vi "GraphForm (SubVI) P.vi"() -> ()   [LabVIEW 2013]
uses:
  Global P.vi
panel:
  out "Sensor 2":dbl format="%.3e"
  out "Sensor 1":dbl format="%.3e"
  in  "P loc":cluster{" P sens 1":dbl, "P sens 2":dbl}
  in  "1_ch_v":bool=TRUE
  in  "stop":bool
  in  "Title":string
  out "часы":string="0"
  in  "Добавить время":dbl(ring)=300.0 items=["1 мин."=60.0, "5 мин."=300.0, "20 мин."=1200.0]
  out "мин.":string="1"
  in  "xScale +":bool
  in  "xScale -":bool
  in  "Autoscale":bool=TRUE
  in  "P max":dbl=0.01 format="%^#.6e"
  in  "P min":dbl=1e-09 format="%^#.6e"
  in  "2_ch_v":bool=TRUE
  in  "T1_col":u32(colorbox)=16448250
  in  "T2_col":u32(colorbox)=2132224
  out "Graphs P":dynamicdata(graph)
  # "P"
  # "[mBar]"
  # "Интервал просмотра"
  # ":"
  # "Шкала P"
  # "P, mBar"
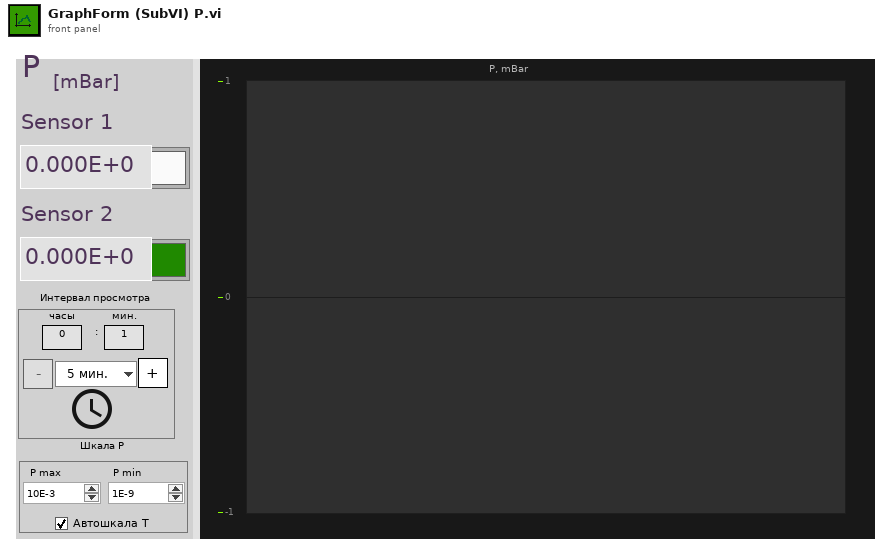
[diagram p1: front panel]
types:
  T1 = typedef "LVDateTimeRec.ctl" = cluster{"fractional second":dbl, "second":i32, "minute":i32, "hour":i32, "day of month":i32, "month":i32, "year":i32, "day of week":i32, "day of year":i32, "DST":i32}
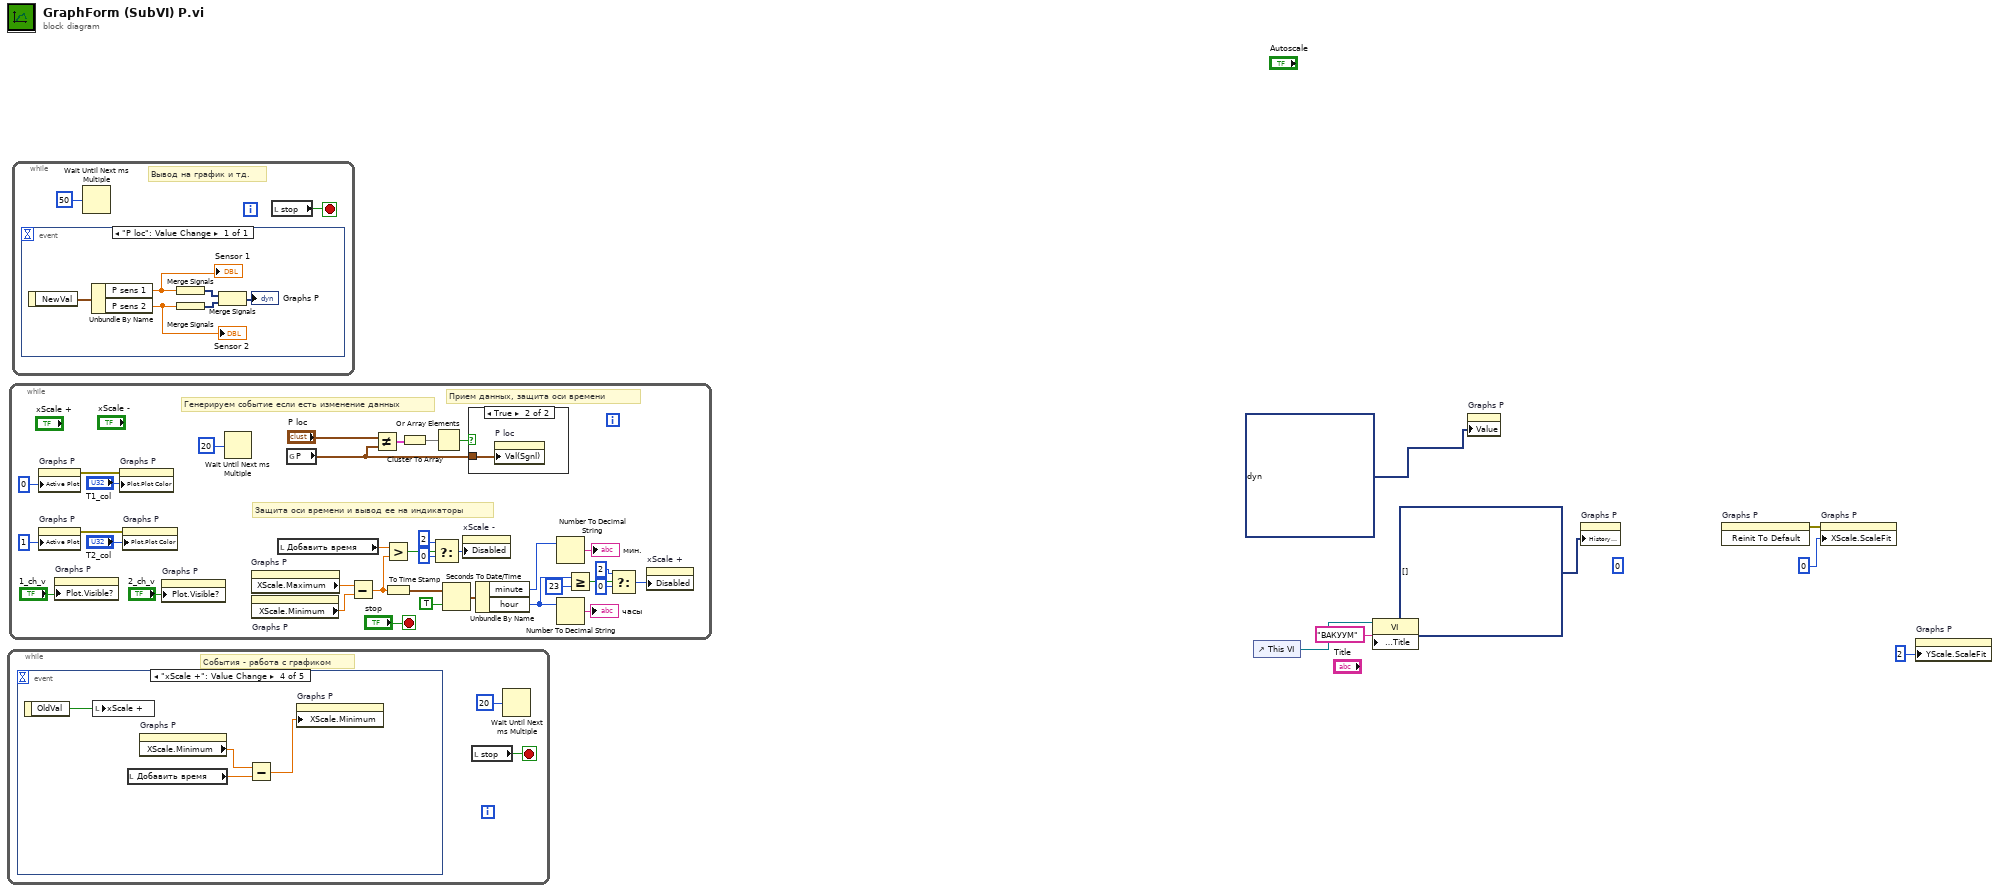
[diagram p0: block diagram]
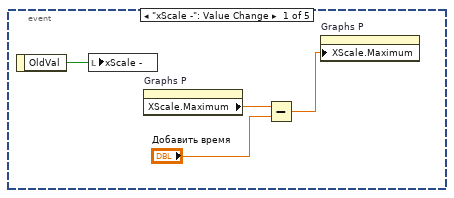
[diagram p3: hidden frame]
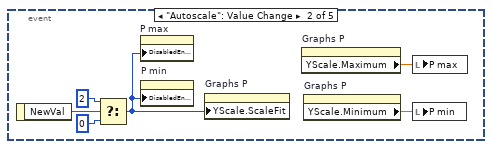
[diagram p4: hidden frame]
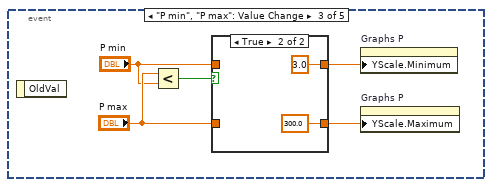
[diagram p5: hidden frame]
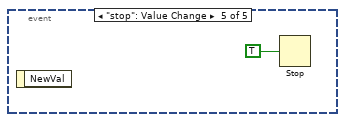
[diagram p7: hidden frame]
diagram:
  (unwired) u8 0 ("Y Scale.Scale Fit")
  n1 = while {
    stop <- w8 stop-if-true
    # "События - работа с графиком"
    n2 = event shown="[3] \"xScale +\": Value Change" {
      selector: _ -> [_ _ _ _ _]
      dyn-events: _ -> [_ _ _ _ _]
      timeout: _ -> [_ _ _ _ _]
      event "xScale -": Value Change {
        n3 = event-data() -> ("OldVal"=w13:bool)  [unwired: 1 out]
        n4 = local write "xScale -"(w13) -> ()
        n5 = property on="Graphs P" class="WFChart (strict)"() -> ("XScale.Maximum"=w11:dbl)  [unwired: 2 in, 2 out]
        n6 = Subtract(x=w11, y="Добавить время") -> (x-y=w12:dbl)
        n7 = property on="Graphs P" class="WFChart (strict)"("XScale.Maximum"=w12) -> ()  [unwired: 2 in, 2 out]
      }
      event "Autoscale": Value Change {
        n8 = event-data() -> ("NewVal"=w14:bool)  [unwired: 1 out]
        n9 = Select(t=u8 2 ("Y Scale.Scale Fit"), s=w14, f=u8 0 ("Y Scale.Scale Fit")) -> (s? t:f=w17:u8)
        n10 = property on="P max" class="DigNum (strict)"("DisabledEnum"=w17) -> ()  [unwired: 2 in, 2 out]
        n11 = property on="P min" class="DigNum (strict)"("DisabledEnum"=w17) -> ()  [unwired: 2 in, 2 out]
        n12 = property on="Graphs P" class="WFChart (strict)"("YScale.ScaleFit"=w17) -> ()  [unwired: 2 in, 2 out]
        n13 = property on="Graphs P" class="WFChart (strict)"() -> ("YScale.Maximum"=w19:dbl)  [unwired: 2 in, 2 out]
        n14 = property on="Graphs P" class="WFChart (strict)"() -> ("YScale.Minimum"=w18:dbl)  [unwired: 2 in, 2 out]
        n15 = local write "P max"(w19) -> ()
        n16 = local write "P min"(w18) -> ()
      }
      event "P min", "P max": Value Change {
        n17 = event-data() -> ()  [unwired: 2 out]
        n18 = Less?(x="P max", y="P min") -> (x < y?=w22:bool)
        n19 = case shown="True" w22 {
          tunnel: [w25 300.0 ("x+1")] -> w24
          tunnel: [w26 3.0 ("x+1")] -> w23
          tunnel: "P max" -> [w25 _]
          tunnel: "P min" -> [w26 _]
          frame False {
          }
          frame True {
          }
        }
        n20 = property on="Graphs P" class="WFChart (strict)"("YScale.Minimum"=w23) -> ()  [unwired: 2 in, 2 out]
        n21 = property on="Graphs P" class="WFChart (strict)"("YScale.Maximum"=w24) -> ()  [unwired: 2 in, 2 out]
      }
      event "xScale +": Value Change {
        n22 = event-data() -> ("OldVal"=w32:bool)  [unwired: 1 out]
        n23 = local write "xScale +"(w32) -> ()
        n24 = local read "Добавить время"() -> (w29:dbl)
        n25 = property on="Graphs P" class="WFChart (strict)"() -> ("XScale.Minimum"=w30:dbl)  [unwired: 2 in, 2 out]
        n26 = Subtract(x=w30, y=w29) -> (x-y=w31:dbl)
        n27 = property on="Graphs P" class="WFChart (strict)"("XScale.Minimum"=w31) -> ()  [unwired: 2 in, 2 out]
      }
      event "stop": Value Change {
        n28 = event-data() -> ()  [unwired: 2 out]
        n29 = Stop(stop? (T)=TRUE) -> ()
      }
    }
    n30 = local read "stop"() -> (w8:bool)
    n31 = Wait Until Next ms Multiple(millisecond multiple=u32 20) -> ()  [unwired: 1 out]
  }
  n32 = while {
    stop <- "stop" stop-if-true
    # "Генерируем событие если есть изменение данных"
    # "Защита оси времени и вывод ее на индикаторы"
    # "Прием данных, защита оси времени"
    n33 = property on="Graphs P" class="WFChart (strict)"("Active Plot"=u32 0) -> (error out=w42:errorcluster)  [unwired: 2 in, 1 out]
    n34 = property on="Graphs P" class="WFChart (strict)"("Active Plot"=u32 1) -> (error out=w44:errorcluster)  [unwired: 2 in, 1 out]
    n35 = property on="Graphs P" class="WFChart (strict)"("Plot.Visible?"="1_ch_v") -> ()  [unwired: 2 in, 2 out]
    n36 = property on="Graphs P" class="WFChart (strict)"(error in=w42, "Plot.Plot Color"="T1_col") -> ()  [unwired: 1 in, 2 out]
    n37 = property on="Graphs P" class="WFChart (strict)"(error in=w44, "Plot.Plot Color"="T2_col") -> ()  [unwired: 1 in, 2 out]
    n38 = property on="Graphs P" class="WFChart (strict)"("Plot.Visible?"="2_ch_v") -> ()  [unwired: 2 in, 2 out]
    n39 = Wait Until Next ms Multiple(millisecond multiple=u32 20) -> ()  [unwired: 1 out]
    n40 = property on="Graphs P" class="WFChart (strict)"() -> ("XScale.Maximum"=w68:dbl)  [unwired: 2 in, 2 out]
    n41 = property on="Graphs P" class="WFChart (strict)"() -> ("XScale.Minimum"=w67:dbl)  [unwired: 2 in, 2 out]
    n42 = local read "Добавить время"() -> (w66:dbl)
    n43 = global read "Global P.vi" "P"() -> (w35:cluster{" P sens 1":dbl, "P sens 2":dbl})
    n44 = Subtract(x=w68, y=w67) -> (x-y=w61:dbl)
    n45 = Not Equal?(x="P loc", y=w35) -> (x != y?=w47:cluster{" P sens 1":bool, "P sens 2":bool})
    n46 = Greater?(x=w66, y=w61) -> (0:w55:bool)
    n47 = To Time Stamp(1:w61) -> (0:w64:timestamp)
    n48 = Cluster To Array(cluster=w47) -> (array=w46:bool[])
    n49 = Select(t=u8 2 ("Disabled"), s=w55, f=u8 0 ("Disabled")) -> (s? t:f=w54:u8)
    n50 = Or Array Elements(Boolean array=w46) -> (logical OR=w45:bool)
    n51 = Seconds To Date/Time(time stamp (now)=w64, to UTC (F)=TRUE) -> (date time rec=w63:T1)
    n52 = property on="xScale -" class="Bool (strict)"("Disabled"=w54) -> ()  [unwired: 2 in, 2 out]
    n53 = case shown="True" w45 {
      tunnel: w35 -> [_ w69]
      frame False {
      }
      frame True {
        n54 = property on="P loc" class="Clust (strict)"("Val(Sgnl)"=w69) -> ()  [unwired: 2 in, 2 out]
      }
    }
    n55 = Unbundle By Name(w63) -> ("minute"=w62:i32, "hour"=w60:i32)
    n56 = Number To Decimal String(number=w62) -> (decimal integer string=→"мин.":string)  [unwired: 1 out]
    n57 = Number To Decimal String(number=w60) -> (decimal integer string=→"часы":string)  [unwired: 1 out]
    n58 = Greater Or Equal?(x=w60, y=23) -> (x >= y?=w50:bool)
    n59 = Select(t=u8 2 ("Disabled"), s=w50, f=u8 0 ("Disabled")) -> (s? t:f=w48:u8)
    n60 = property on="xScale +" class="Bool (strict)"("Disabled"=w48) -> ()  [unwired: 2 in, 2 out]
  }
  n61 = while {
    stop <- w70 stop-if-true
    # "Вывод на график и тд."
    n62 = event shown="[0] \"P loc\": Value Change" {
      selector: _ -> [_]
      dyn-events: _ -> [_]
      timeout: _ -> [_]
      event "P loc": Value Change {
        n63 = event-data() -> ("NewVal"=w74:cluster{" P sens 1":dbl, "P sens 2":dbl})  [unwired: 1 out]
        n64 = Unbundle By Name(w74) -> ("P sens 1"=w73:dbl, "P sens 2"=w72:dbl)
        "Sensor 1" <- w73
        "Sensor 2" <- w72
        n65 = Merge Signals(w73) -> (w77:dynamicdata)
        n66 = Merge Signals(w72) -> (w76:dynamicdata)
        n67 = Merge Signals(w77, w76) -> (→"Graphs P":dynamicdata)
      }
    }
    n68 = Wait Until Next ms Multiple(millisecond multiple=u32 50) -> ()  [unwired: 1 out]
    n69 = local read "stop"() -> (w70:bool)
  }
  n70 = control-ref of="This VI"() -> (w2:refnum<vi>)
  n71 = property class="VI"(reference=w2, "Front Panel.Title"="ВАКУУМ" ("Front Panel Window:Title")) -> ()  [unwired: 1 in, 2 out]
  n72 = property on="Graphs P" class="WFChart (strict)"("Value"=dynamicdata [{"t0"=timestamp(3465273261.7246556 s since 1904-01-01), "dt"=1.0, "Y"=[0.1931097262457384]}, {"t0"=timestamp(3465273261.7246556 s since 1904-01-01), "dt"=1.0, "Y"=[0.3594116459482981]}, {"t0"=timestamp(3465273261.7246556 s since 1904-01-01), "dt"=1.0, "Y"=[0.8898205452798131]}, {"t0"=timestamp(3465273261.7246556 s since 1904-01-01), "dt"=1.0, "Y"=[0.747699236883661]}] ("Graphs")) -> ()  [unwired: 2 in, 2 out]
  n73 = property on="Graphs P" class="WFChart (strict)"("History Data"=dynamicdata[] []) -> ()  [unwired: 2 in, 2 out]
  n74 = invoke on="Graphs P" class="WFChart (strict)" method="Reinit To Default"() -> (error out=w4:errorcluster)  [unwired: 3 in, 2 out]
  n75 = property on="Graphs P" class="WFChart (strict)"(error in=w4, "XScale.ScaleFit"=u8 0 ("Y Scale.Scale Fit")) -> ()  [unwired: 1 in, 2 out]
  n76 = property on="Graphs P" class="WFChart (strict)"("YScale.ScaleFit"=u8 2 ("Y Scale.Scale Fit")) -> ()  [unwired: 2 in, 2 out]
